vi "sub_cal_pcb_temp.vi"(11 "ir temp":dbl[][](array[numeric])) -> (3 "pcb temp":dbl[][](array[numeric]))   [LabVIEW 2016]
uses:
  <vilib>/Analysis/NI_AALPro.lvlib
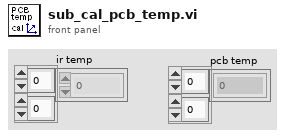
[diagram p1: front panel]
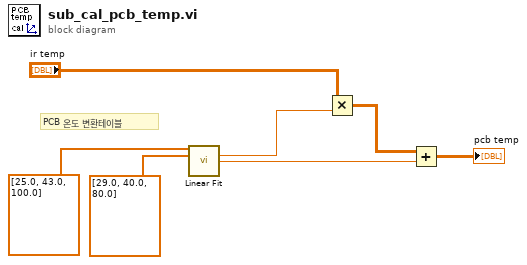
[diagram p0: block diagram]
diagram:
  # "PCB 온도 변환테이블"
  n1 = call <vilib>:"Linear Fit.vi"("Y"=dbl[] [25.0, 43.0, 100.0] ("X"), "X"=dbl[] [29.0, 40.0, 80.0]) -> ("slope"=w1:dbl, "intercept"=w4:dbl)  [unwired: 9 in, 3 out]
  n2 = Multiply(x="ir temp", y=w1) -> (x*y=w5:dbl[][])
  n3 = Add(x=w5, y=w4) -> (x+y=→"pcb temp":dbl[][])
